vi "ui_DataLog Query Listed Strings.vi"(0 "prompt":string, 7 "list of strings":string[](array[string])) -> (4 "OKed?":bool, 8 "selected strings":string[](array[string]))   [LabVIEW 2012]
doc: "Allows a set of strings to be easily selected from a list of candidate strings. The titlebar displays the prompt that explains what is in need of being selected. It is pick strings from the list, type the first part of the string to reduce the list of candidates, or to specify a subset via the '?' and '*' wildcards."
uses:
  typedefs/t_DataLog Query Listed Strings States.ctl
panel:
  in  "none":bool
  in  "all":bool
  in  "pattern":string
  in  "list":i32(listbox)
  in  "cancel":bool
  in  "OK":bool
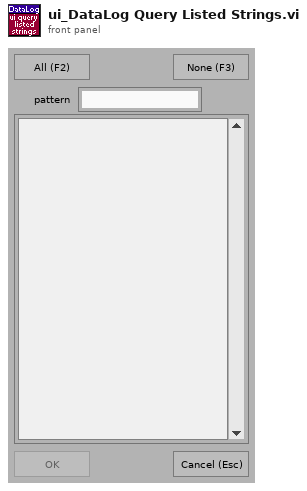
[diagram p1: front panel]
types:
  T1 = typedef "t_DataLog Query Listed Strings States.ctl" = enum16{"empty queue", "select", "filter list", "ablement", "initialize", "init controls", "init check list", "init filter", "cleanup", "stop"}
  T2 = typedef "eventvkey.ctl" = enum16{"ASCII", "Enter", "Return", "Shift", "Ctrl", "Alt", "Cmd", "Opt", "Caps", "NumLock", "Clear", "Break", "Up", "Down", "Left", "Right", "Insert", "Delete", "Home", "End", "PageUp", "PageDown", "Escape", "Help", "Pause", "ScrollLock", "F1", "F2", "F3", "F4", "F5", "F6", "F7", "F8", "F9", "F10", "F11", "F12", "F13", "F14", "F15", "F16", "F17", "F18", "F19", "F20", "F21", "F22", "F23", "F24", "Play", "VolumeUp", "VolumeDown", "Mute", "Two Byte Char"}
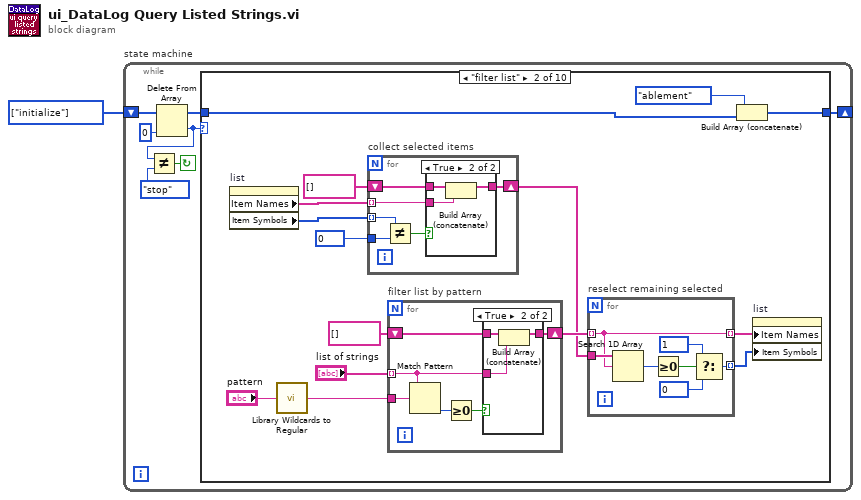
[diagram p0: block diagram]
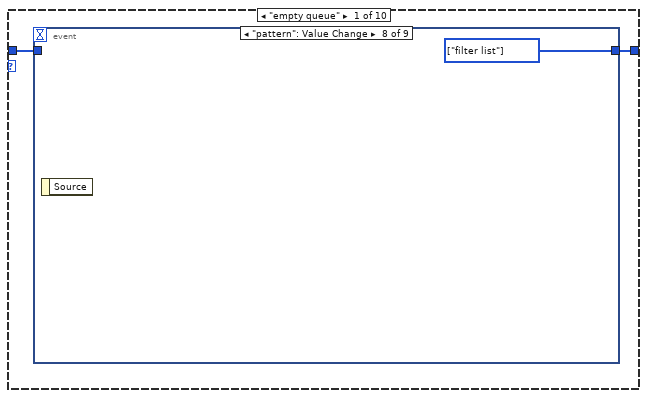
[diagram p2: hidden frame]
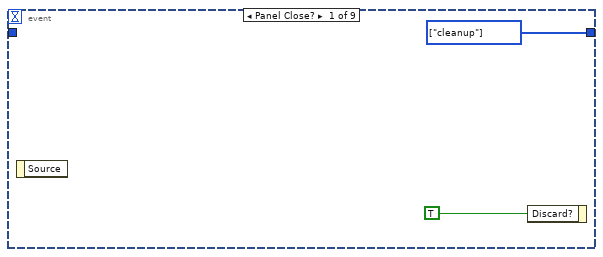
[diagram p3: hidden frame]
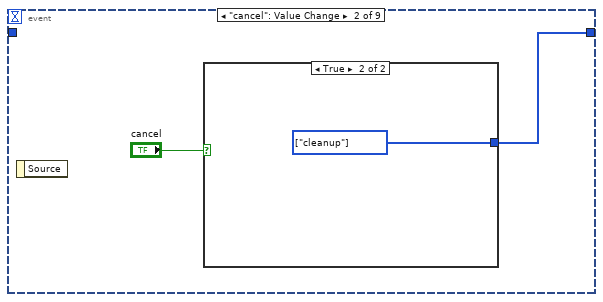
[diagram p4: hidden frame]
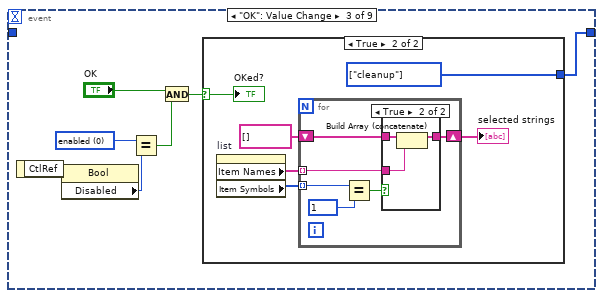
[diagram p6: hidden frame]
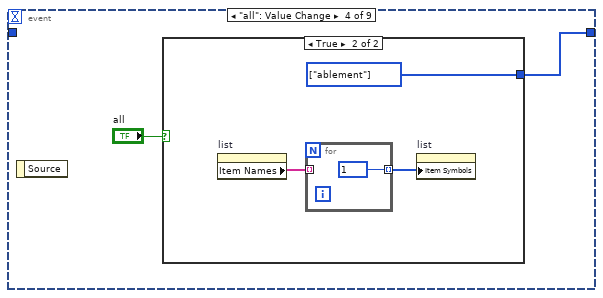
[diagram p9: hidden frame]
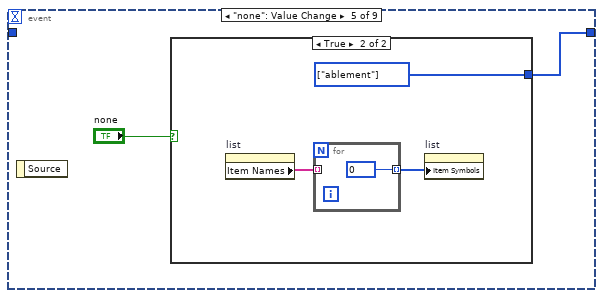
[diagram p11: hidden frame]
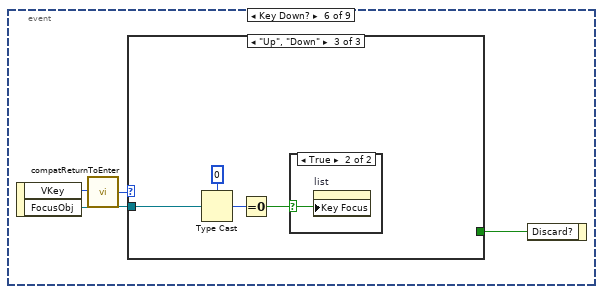
[diagram p13: hidden frame]
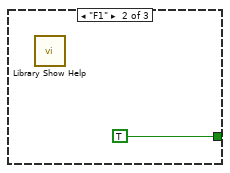
[diagram p15: hidden frame]
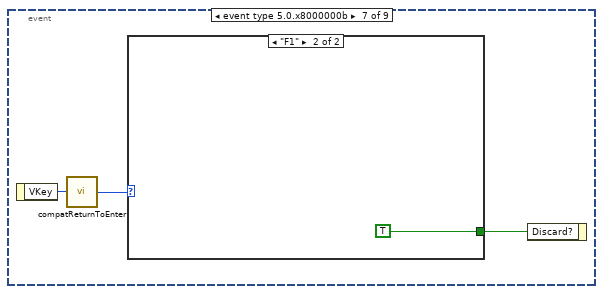
[diagram p17: hidden frame]
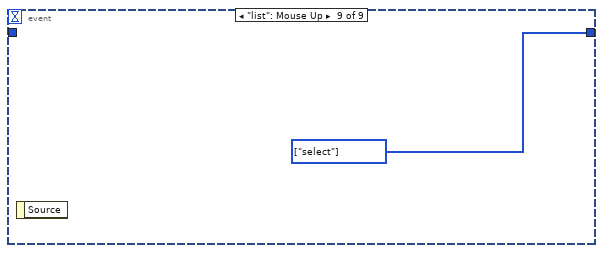
[diagram p19: hidden frame]
diagram:
  w1 = T1[] [enum."initialize"] items=["empty queue", "select", "filter list", "ablement", "initialize", "init controls", "init check list", "init filter", "cleanup", "stop"] ("Array Constant")
  n1 = while "state machine" {
    shift-left: w1 -> [w5]
    shift-right: [w8] -> _
    stop <- w7 continue-if-true
    n2 = Delete From Array(array=w5, index=0) -> (deleted portion=w2:T1, array with subset deleted=w4:T1[])  [unwired: 1 in]
    n3 = Not Equal?(x=w2, y=t_DataLog_Query_Listed_Strings_States."stop" ("states")) -> (x != y?=w7:bool)
    n4 = case "Case" shown="\"filter list\"" w2 {
      tunnel: [w10 w77 w110 w126 w132 w164 w165 w172 w177 w178] -> w8
      tunnel: w4 -> [w9 w76 w109 w126 _ w164 w166 w173 _ w178]
      frame "empty queue" {
        n5 = event shown="[7] \"pattern\": Value Change" {
          selector: _ -> [_ _ _ _ _ _ _ _ _]
          dyn-events: _ -> [_ _ _ _ _ _ _ _ _]
          timeout: _ -> [_ _ _ _ _ _ _ _ _]
          tunnel: [w12 w13 w22 w40 w46 _ _ w65 w66] -> w10
          tunnel: w9 -> [_ _ _ _ _ _ _ _ _]
          event Panel Close? {
            w12 = T1[] [enum."cleanup"] items=["empty queue", "select", "filter list", "ablement", "initialize", "init controls", "init check list", "init filter", "cleanup", "stop"] ("Array Constant")
            n6 = event-data() -> ()  [unwired: 1 in, 1 out]
            n7 = event-data("Discard?"=TRUE) -> ()  [unwired: 1 in, 1 out]
          }
          event "cancel": Value Change {
            n8 = event-data() -> ()  [unwired: 1 in, 1 out]
            n9 = case shown="True" "cancel" {
              tunnel: [_ w15] -> w13
              frame False {
              }
              frame True {
                w15 = T1[] [enum."cleanup"] items=["empty queue", "select", "filter list", "ablement", "initialize", "init controls", "init check list", "init filter", "cleanup", "stop"] ("Array Constant")
              }
            }
          }
          event "OK": Value Change {
            w19 = u8 0 items=["enabled", "disabled", "grayed"] ("disabled state")
            n10 = event-data() -> ("CtlRef"=w21:refnum<vi>)  [unwired: 1 in]
            n11 = property class="Bool"(reference=w21) -> ("Disabled"=w20:u8)  [unwired: 1 in, 2 out]
            n12 = Equal?(x=w19, y=w20) -> (x = y?=w18:bool)
            n13 = And(x="OK", y=w18) -> (x .and. y?=w17:bool)
            n14 = case shown="True" w17 {
              selector: w17 -> [_ w27]
              tunnel: [_ w28] -> w22
              frame False {
              }
              frame True {
                w28 = T1[] [enum."cleanup"] items=["empty queue", "select", "filter list", "ablement", "initialize", "init controls", "init check list", "init filter", "cleanup", "stop"] ("Array Constant")
                n15 = property on="list" class="LstBox (strict)"() -> ("Item Names"=w26:string[], "Item Symbols"=w25:i32[])  [unwired: 2 in, 2 out]
                n16 = for {
                  tunnel: w26 -> [w30] mode=indexing
                  tunnel: w25 -> [w34] mode=indexing
                  shift-right: [w29] -> w24
                  shift-left: string[] [] -> [w31]
                  n17 = Equal?(x=w34, y=1) -> (x = y?=w32:bool)
                  n18 = case shown="True" w32 {
                    tunnel: w31 -> [w35 w38]
                    tunnel: w30 -> [_ w37]
                    tunnel: [w35 w36] -> w29
                    frame False {
                    }
                    frame True {
                      n19 = Build Array (concatenate)(w38, w37) -> (w36:string[])
                    }
                  }
                }
                "selected strings" <- w24
                "OKed?" <- w27
              }
            }
          }
          event "all": Value Change {
            n20 = event-data() -> ()  [unwired: 1 in, 1 out]
            n21 = case shown="True" "all" {
              tunnel: [_ w43] -> w40
              frame False {
              }
              frame True {
                w43 = T1[] [enum."ablement"] items=["empty queue", "select", "filter list", "ablement", "initialize", "init controls", "init check list", "init filter", "cleanup", "stop"] ("Array Constant")
                n22 = property on="list" class="LstBox (strict)"() -> ("Item Names"=w42:string[])  [unwired: 2 in, 2 out]
                n23 = for {
                  tunnel: w42 -> [_] mode=indexing
                  tunnel: [1] -> w41 mode=indexing
                }
                n24 = property on="list" class="LstBox (strict)"("Item Symbols"=w41) -> ()  [unwired: 2 in, 2 out]
              }
            }
          }
          event "none": Value Change {
            n25 = event-data() -> ()  [unwired: 1 in, 1 out]
            n26 = case shown="True" "none" {
              tunnel: [_ w49] -> w46
              frame False {
              }
              frame True {
                w49 = T1[] [enum."ablement"] items=["empty queue", "select", "filter list", "ablement", "initialize", "init controls", "init check list", "init filter", "cleanup", "stop"] ("Array Constant")
                n27 = property on="list" class="LstBox (strict)"() -> ("Item Names"=w48:string[])  [unwired: 2 in, 2 out]
                n28 = for {
                  tunnel: w48 -> [_] mode=indexing
                  tunnel: [0] -> w47 mode=indexing
                }
                n29 = property on="list" class="LstBox (strict)"("Item Symbols"=w47) -> ()  [unwired: 2 in, 2 out]
              }
            }
          }
          event Key Down? {
            n30 = event-data() -> ("VKey"=w51:T2, "FocusObj"=w52:refnum<vi>)  [unwired: 1 in]
            n31 = call <vilib>:"compatReturnToEnter.vi"("VKey"=w51) -> ("VKey"=w54:T2)
            n32 = case shown="\"Up\", \"Down\"" w54 {
              tunnel: [_ TRUE ("Discard?") _] -> w53
              tunnel: w52 -> [_ _ w57]
              frame Default {
              }
              frame "F1" {
                n33 = call "Library Show Help.vi"() -> ()  [unwired: 1 in]
              }
              frame "Up", "Down" {
                n34 = Type Cast(type=0, x=w57) -> (*(type *) &x=w59:i32)
                n35 = Equal To 0?(x=w59) -> (x = 0?=w56:bool)
                n36 = case shown="True" w56 {
                  selector: w56 -> [_ w60]
                  frame False {
                  }
                  frame True {
                    n37 = property on="list" class="LstBox (strict)"("Key Focus"=w60) -> ()  [unwired: 2 in, 2 out]
                  }
                }
              }
            }
            n38 = event-data("Discard?"=w53) -> ()  [unwired: 1 in, 1 out]
          }
          event event type 5.0.x8000000b {
            n39 = event-data() -> ("VKey"=w61:T2)  [unwired: 1 in]
            n40 = call <vilib>:"compatReturnToEnter.vi"("VKey"=w61) -> ("VKey"=w63:T2)
            n41 = case shown="\"F1\"" w63 {
              tunnel: [_ TRUE ("Discard?")] -> w62
              frame Default {
              }
              frame "F1" {
              }
            }
            n42 = event-data("Discard?"=w62) -> ()  [unwired: 1 in, 1 out]
          }
          event "pattern": Value Change {
            w65 = T1[] [enum."filter list"] items=["empty queue", "select", "filter list", "ablement", "initialize", "init controls", "init check list", "init filter", "cleanup", "stop"] ("Array Constant")
            n43 = event-data() -> ()  [unwired: 1 in, 1 out]
          }
          event "list": Mouse Up {
            w66 = T1[] [enum."select"] items=["empty queue", "select", "filter list", "ablement", "initialize", "init controls", "init check list", "init filter", "cleanup", "stop"] ("Array Constant")
            n44 = event-data() -> ()  [unwired: 1 in, 1 out]
          }
        }
      }
      frame "filter list" {
        n45 = property on="list" class="LstBox (strict)"() -> ("Item Names"=w75:string[], "Item Symbols"=w74:i32[])  [unwired: 2 in, 2 out]
        n46 = call "Library Wildcards to Regular.vi"("wildcards"="pattern") -> ("regular expression"=w67:string)  [unwired: 4 in]
        n47 = for "collect selected items" {
          tunnel: w75 -> [w91] mode=indexing
          tunnel: w74 -> [w94] mode=indexing
          tunnel: 0 -> [w93]
          shift-right: [w89] -> w69
          shift-left: string[] [] -> [w90]
          n48 = Not Equal?(x=w94, y=w93) -> (x != y?=w92:bool)
          n49 = case shown="True" w92 {
            tunnel: w91 -> [_ w98]
            tunnel: w90 -> [w95 w97]
            tunnel: [w95 w96] -> w89
            frame False {
            }
            frame True {
              n50 = Build Array (concatenate)(w97, w98) -> (w96:string[])
            }
          }
        }
        n51 = for "filter list by pattern" {
          tunnel: w67 -> [w104]
          tunnel: "list of strings" -> [w101] mode=indexing
          shift-right: [w99] -> w71
          shift-left: string[] [] -> [w100]
          n52 = Match Pattern(string=w101, regular expression=w104) -> (offset past match=w103:i32)  [unwired: 1 in, 3 out]
          n53 = Greater Or Equal To 0?(x=w103) -> (x >= 0?=w102:bool)
          n54 = case shown="True" w102 {
            tunnel: w101 -> [_ w108]
            tunnel: w100 -> [w105 w107]
            tunnel: [w105 w106] -> w99
            frame False {
            }
            frame True {
              n55 = Build Array (concatenate)(w107, w108) -> (w106:string[])
            }
          }
        }
        n56 = for "reselect remaining selected" {
          tunnel: w71 -> [w87] mode=indexing
          tunnel: [w87] -> w70 mode=indexing
          tunnel: w69 -> [w88]
          tunnel: [w82] -> w68 mode=indexing
          n57 = Search 1D Array(1D array=w88, element=w87) -> (index of element=w86:i32)  [unwired: 1 in]
          n58 = Greater Or Equal To 0?(x=w86) -> (x >= 0?=w85:bool)
          n59 = Select(t=1, s=w85, f=0) -> (s? t:f=w82:i32)
        }
        n60 = Build Array (concatenate)(t_DataLog_Query_Listed_Strings_States."ablement" ("states"), w76) -> (w77:T1[])
        n61 = property on="list" class="LstBox (strict)"("Item Names"=w70, "Item Symbols"=w68) -> ()  [unwired: 2 in, 2 out]
      }
      frame "select" {
        w117 = 0
        n62 = property on="list" class="LstBox (strict)"() -> ("Item Symbols"=w119:i32[])  [unwired: 2 in, 2 out]
        n63 = Index Array(array=w119, index="list") -> (element=w115:i32)
        n64 = Equal?(x=w115, y=w117) -> (x = y?=w118:bool)
        n65 = Select(t=1, s=w118, f=w117) -> (s? t:f=w114:i32)
        n66 = Replace Array Subset(array=w119, new element=w114, index="list") -> (w113:i32[])
        n67 = property on="list" class="LstBox (strict)"("Item Symbols"=w113) -> ()  [unwired: 2 in, 2 out]
        n68 = Build Array (concatenate)(t_DataLog_Query_Listed_Strings_States."ablement" ("states"), w109) -> (w110:T1[])
      }
      frame "ablement" {
        w121 = u8 2 items=["enabled", "disabled", "grayed"] ("disabled state")
        w122 = u8 0 items=["enabled", "disabled", "grayed"] ("disabled state")
        n69 = property on="list" class="LstBox (strict)"() -> ("Item Symbols"=w125:i32[])  [unwired: 2 in, 2 out]
        n70 = for {
          tunnel: w125 -> [w131] mode=indexing
          shift-right: [w127] -> w123
          shift-left: FALSE -> [w129]
          n71 = Not Equal?(x=0, y=w131) -> (x != y?=w128:bool)
          n72 = Or(x=w128, y=w129) -> (x .or. y?=w127:bool)
        }
        n73 = Select(t=w122, s=w123, f=w121) -> (s? t:f=w120:u8)
        n74 = property on="OK" class="Bool"("Disabled"=w120) -> ()  [unwired: 2 in, 2 out]
      }
      frame "initialize" {
        n75 = while "rebuild init list on first run or after load or recompile" {
          shift-left: _ -> [w135]
          shift-right: [w134] -> w132
          stop <- FALSE continue-if-true
          n76 = Array Size(array=w135) -> (size(s)=w136:i32)
          n77 = case shown="0" w136 {
            tunnel: [w137 w157] -> w134
            tunnel: w135 -> [w138 w157]
            frame 0 {
              n78 = while {
                shift-left: w138 -> [w147]
                shift-right: [w145] -> w137
                shift-left: _ -> [w149]
                shift-right: [w144] -> _
                i -> [w152]
                stop <- w140 continue-if-true
                n79 = To Unsigned Word Integer(number=w152) -> (unsigned 16bit integer=w150:u16)
                n80 = Type Cast(type=t_DataLog_Query_Listed_Strings_States."initialize" ("states"), x=w150) -> (*(type *) &x=w146:T1)
                n81 = Format Into String(format string="%s" ("Format String"), w146) -> (resulting string=w144:string)  [unwired: 2 in, 1 out]
                n82 = Not Equal?(x=w144, y=w149) -> (x != y?=w140:bool)
                n83 = Match Pattern(string=w144, regular expression="^init ") -> (offset past match=w142:i32)  [unwired: 1 in, 3 out]
                n84 = Greater Or Equal To 0?(x=w142) -> (x >= 0?=w141:bool)
                n85 = And(x=w141, y=w140) -> (x .and. y?=w139:bool)
                n86 = case shown="True" w139 {
                  tunnel: w147 -> [w153 w156]
                  tunnel: w146 -> [_ w155]
                  tunnel: [w153 w154] -> w145
                  frame False {
                  }
                  frame True {
                    n87 = Build Array (concatenate)(w156, w155) -> (w154:T1[])
                  }
                }
              }
            }
            frame Default {
            }
          }
        }
      }
      frame "init controls" {
        n88 = local write "selected strings"(string[] [] ("selected strings")) -> ()
        n89 = local write "OKed?"(FALSE ("OKed?")) -> ()
        n90 = property on="pattern" class="Str"("Key Focus"=TRUE, "Value"="*") -> ()  [unwired: 2 in, 2 out]
        n91 = local write "list"(-1 ("list")) -> ()
        n92 = property class="VI"("Front Panel Window:Title"="prompt") -> ()  [unwired: 2 in, 2 out]
      }
      frame "init check list" {
        w167 = T1[] [enum."stop"] items=["empty queue", "select", "filter list", "ablement", "initialize", "init controls", "init check list", "init filter", "cleanup", "stop"] ("Array Constant")
        n93 = local read "list of strings"() -> (w170:string[])
        n94 = Array Size(array=w170) -> (size(s)=w169:i32)
        n95 = Not Equal To 0?(x=w169) -> (x != 0?=w168:bool)
        n96 = Select(t=w166, s=w168, f=w167) -> (s? t:f=w165:T1[])
      }
      frame "init filter" {
        n97 = Build Array (concatenate)(t_DataLog_Query_Listed_Strings_States."filter list" ("states"), w173) -> (w172:T1[])
      }
      frame "cleanup" {
        w175 = u8 2 items=["enabled", "disabled", "grayed"] ("disabled state")
        w177 = T1[] [enum."stop"] items=["empty queue", "select", "filter list", "ablement", "initialize", "init controls", "init check list", "init filter", "cleanup", "stop"] ("Array Constant")
        n98 = local write "pattern"("" ("pattern")) -> ()
        n99 = property on="list" class="LstBox (strict)"("Item Names"=string[] []) -> ()  [unwired: 2 in, 2 out]
        n100 = property on="OK" class="Bool"("Disabled"=w175) -> ()  [unwired: 2 in, 2 out]
      }
      frame "stop" {
      }
    }
  }
